vi "draw_circle_image.vi"(1 "Color":u32(colorbox)=16711680, 2 "radius":dbl format="%#_13g", 3 "Position":cluster{"X":sgl, "Y":sgl}, 4 "Image":T1) -> (0 "Image Out":T1)   [LabVIEW 2018]
uses:
  <vilib>/vision/Image Controls.llb/IMAQ Image.ctl
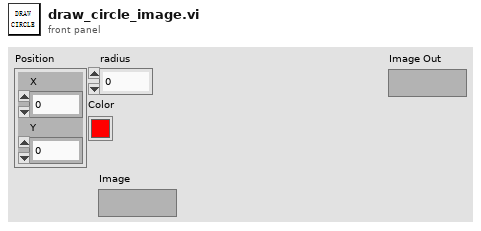
[diagram p1: front panel]
types:
  T1 = typedef "IMAQ Image.ctl" = refnum<image>
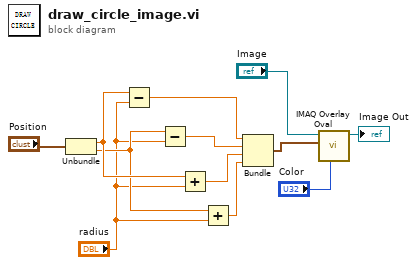
[diagram p0: block diagram]
diagram:
  n1 = Unbundle("Position") -> ("X"=w11:sgl, "Y"=w10:sgl)
  n2 = Subtract(x=w11, y="radius") -> (x-y=w8:dbl)
  n3 = Subtract(x=w10, y="radius") -> (x-y=w7:dbl)
  n4 = Add(x=w11, y="radius") -> (x+y=w6:dbl)
  n5 = Add(x=w10, y="radius") -> (x+y=w5:dbl)
  n6 = Bundle(w8, w7, w6, w5) -> (w4:cluster{dbl, dbl, dbl, dbl})  [unwired: 1 in]
  n7 = call "IMAQ Overlay Oval"("Color"="Color", "Bounding Rectangle"=w4, "Image"="Image") -> ("Image Out"=→"Image Out":T1)  [unwired: 7 in, 1 out]
